vi "tape.fitness02_SS.vi"(2 "New Image":T2=refnum) -> ()   [LabVIEW 2013]
uses:
  <vilib>/vision/Image Controls.llb/IMAQ Image.ctl
  <vilib>/vision/NI_Vision_Development_Module.lvlib
panel:
  out "x/y 2":sgl
  out "x/y":sgl
  out "Waveform Chart 4":sgl(graph)=1.0503659
  out "In Range? 2":bool=TRUE
  in  "upper limit 2":sgl=1.1
  in  "lower  limit 2":sgl=0.9
  in  "Boolean":bool
  in  "Settings 2":T1={"Contrast"=170, "Filter width"=4, "Steepness"=50, "Subsampling Ratio"=10.0, "Scan Direction"=1, "Show Search Area"=TRUE, "Show Search Lines"=FALSE, "Show Edges Found"=TRUE, "Show Result"=TRUE} {"Scan Direction" items=["Outside to Inside", "Inside to Outside"]}
  in  "shot number":i16
  in  "lower  limit":sgl=0.9
  in  "upper limit":sgl=1.1
  out "In Range?":bool=TRUE
  out "Waveform Chart 3":sgl(graph)=1.0234288
  out "Y Graph":cluster{i16, "Y":sgl}[](graph)=[{1, "Y"=174.77158}, {1, "Y"=173.48274}, {1, "Y"=268.76178}, {1, "Y"=279.66354}]
  out "X Graph":cluster{i16, "X":sgl}[](graph)=[{1, "X"=246.72554}, {1, "X"=149.21423}, {1, "X"=152.1977}, {1, "X"=252.06}]
  out "tape status":bool=TRUE
  out "XY Graph":cluster{"X":sgl, "Y":sgl}[](graph)=[{"X"=246.72554, "Y"=174.77158}, {"X"=149.21423, "Y"=173.48274}, {"X"=152.1977, "Y"=268.76178}, {"X"=252.06, "Y"=279.66354}]
  out "Radius":dbl=52.693813240488524
  in  "Location of structure":T3={"Center X"=198, "Center Y"=228, "Inner Radius"=0, "Outer Radius"=210, "Start Angle"=0.0, "End Angle"=0.0} {"End Angle" format="%.2f"; "Start Angle" format="%.2f"; "Center X" scale=0.0..1024.0}
  in  "Settings":T1={"Contrast"=170, "Filter width"=4, "Steepness"=9, "Subsampling Ratio"=10.0, "Scan Direction"=1, "Show Search Area"=TRUE, "Show Search Lines"=FALSE, "Show Edges Found"=TRUE, "Show Result"=TRUE} {"Scan Direction" items=["Outside to Inside", "Inside to Outside"]}
  in  "input anulus 2":T3={"Center X"=173, "Center Y"=143, "Inner Radius"=0, "Outer Radius"=57, "Start Angle"=0.0, "End Angle"=0.0} {"End Angle" min=-90.0 max=90.0 step=1.0 format="%.2f"; "Start Angle" min=-90.0 max=90.0 step=1.0 format="%.2f"; "Center X" scale=0.0..1024.0}
  out "Image":T2(plugin-control)
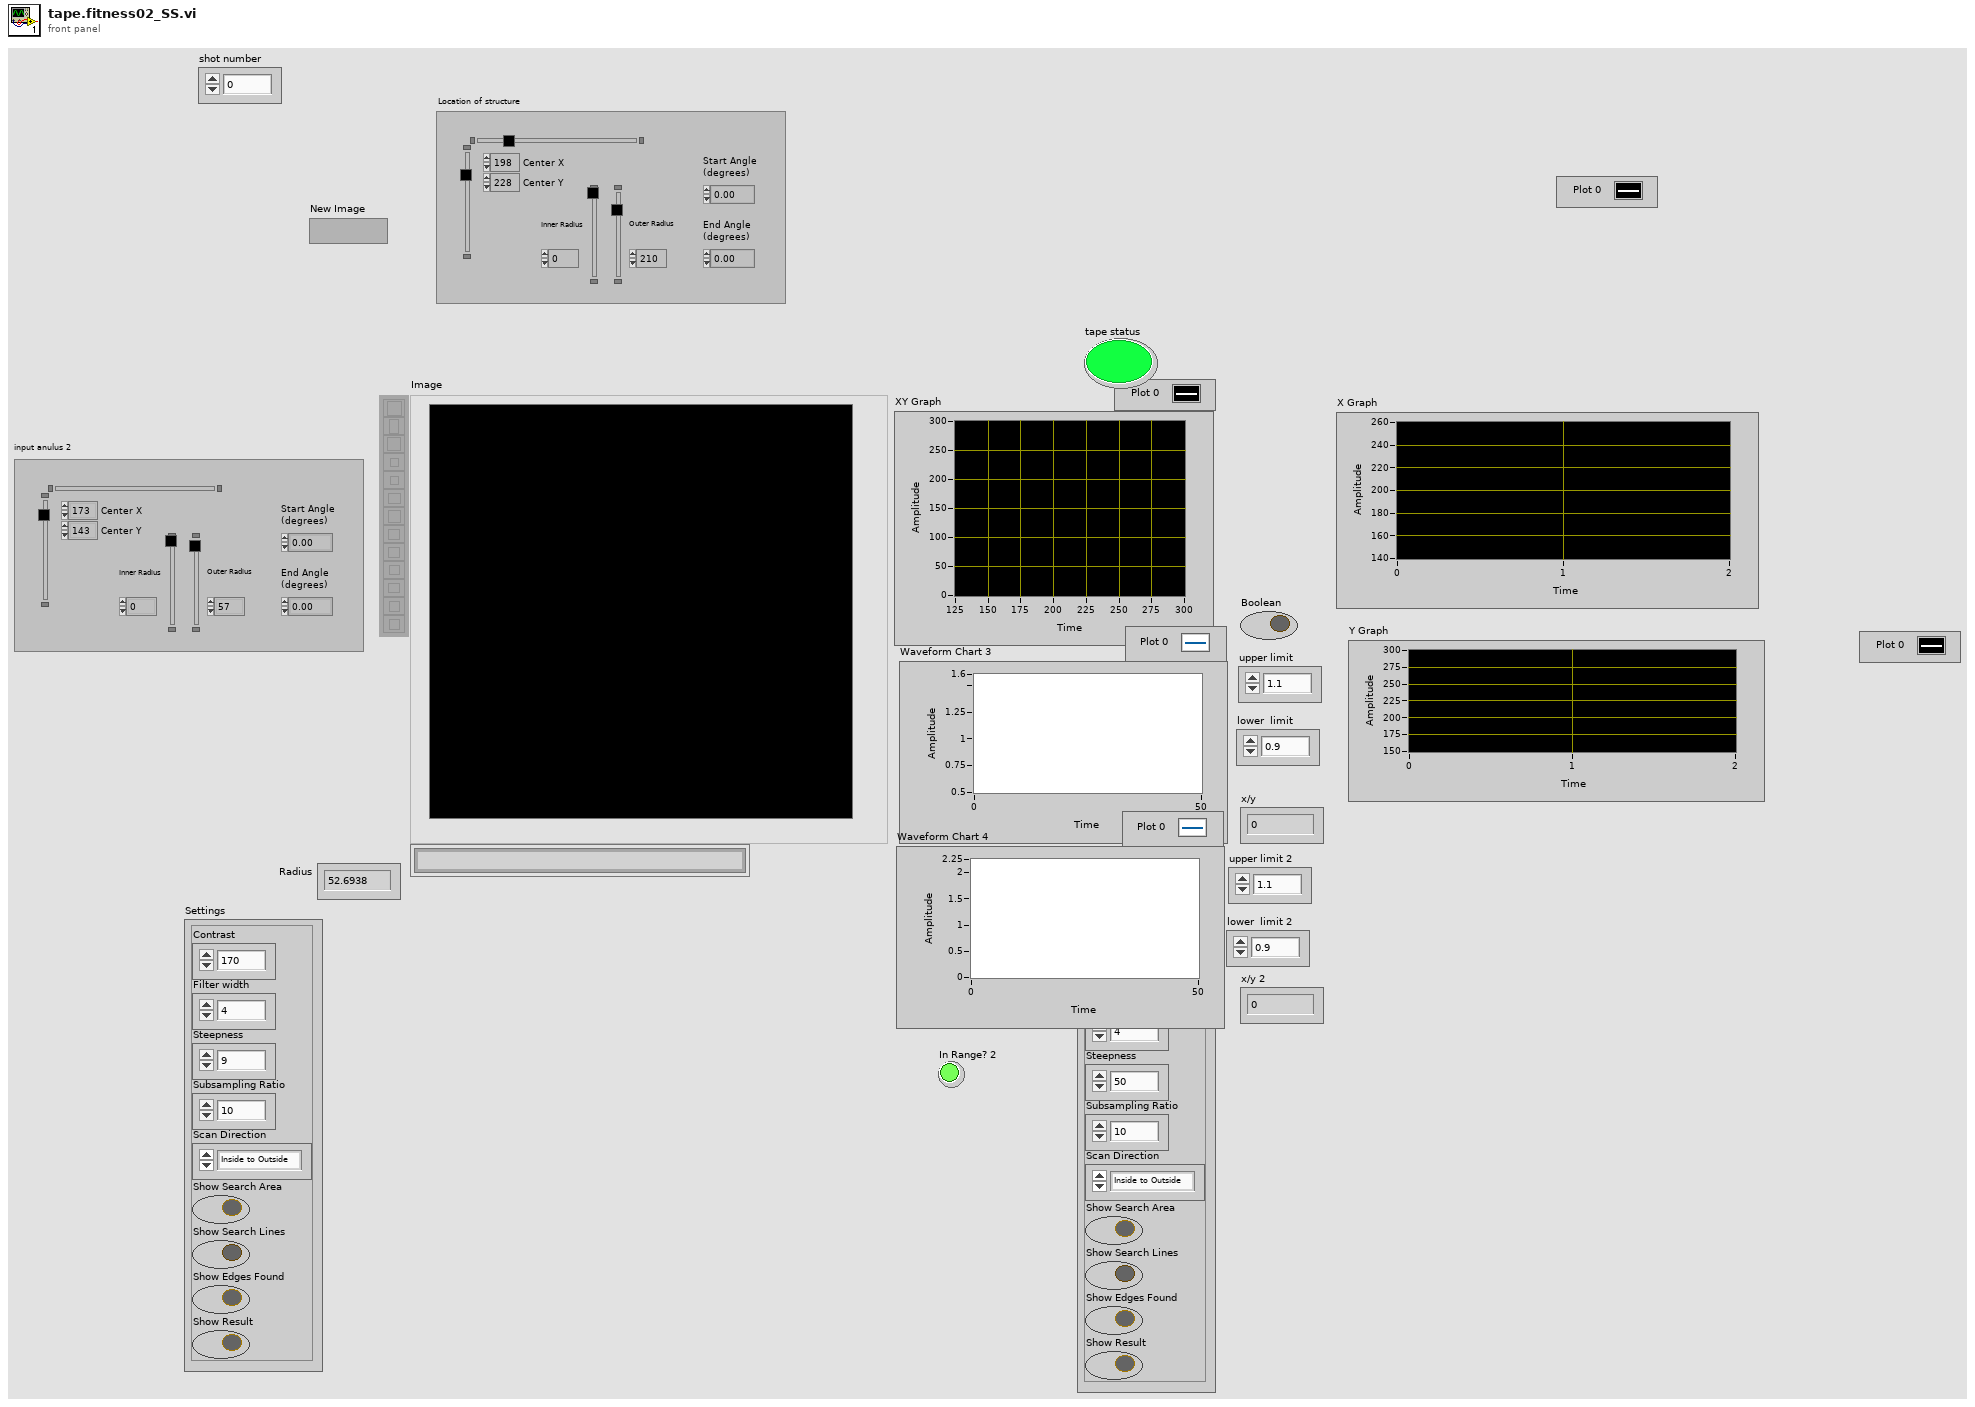
[diagram p1: front panel]
types:
  T1 = cluster{"Contrast":i32, "Filter width":i32, "Steepness":i32, "Subsampling Ratio":dbl, "Scan Direction":u32, "Show Search Area":bool, "Show Search Lines":bool, "Show Edges Found":bool, "Show Result":bool}
  T2 = typedef "IMAQ Image.ctl" = refnum<image>
  T3 = typedef "IMAQ Circle" = cluster{"Center X":i32, "Center Y":i32, "Inner Radius":i32, "Outer Radius":i32, "Start Angle":dbl, "End Angle":dbl}
  T4 = cluster{"Global Rectangle":i32[], "Contours":cluster{"Contour Type":u32, "ROI Type":u32, "Points":i32[]}[]}
  T5 = cluster{"Contour Type":u32, "ROI Type":u32, "Points":i32[]}[]
  T6 = cluster{"Contour Type":u32, "ROI Type":u32, "Points":i32[]}
  T7 = cluster{"Center":cluster{"X":sgl, "Y":sgl}, "Radius":dbl}
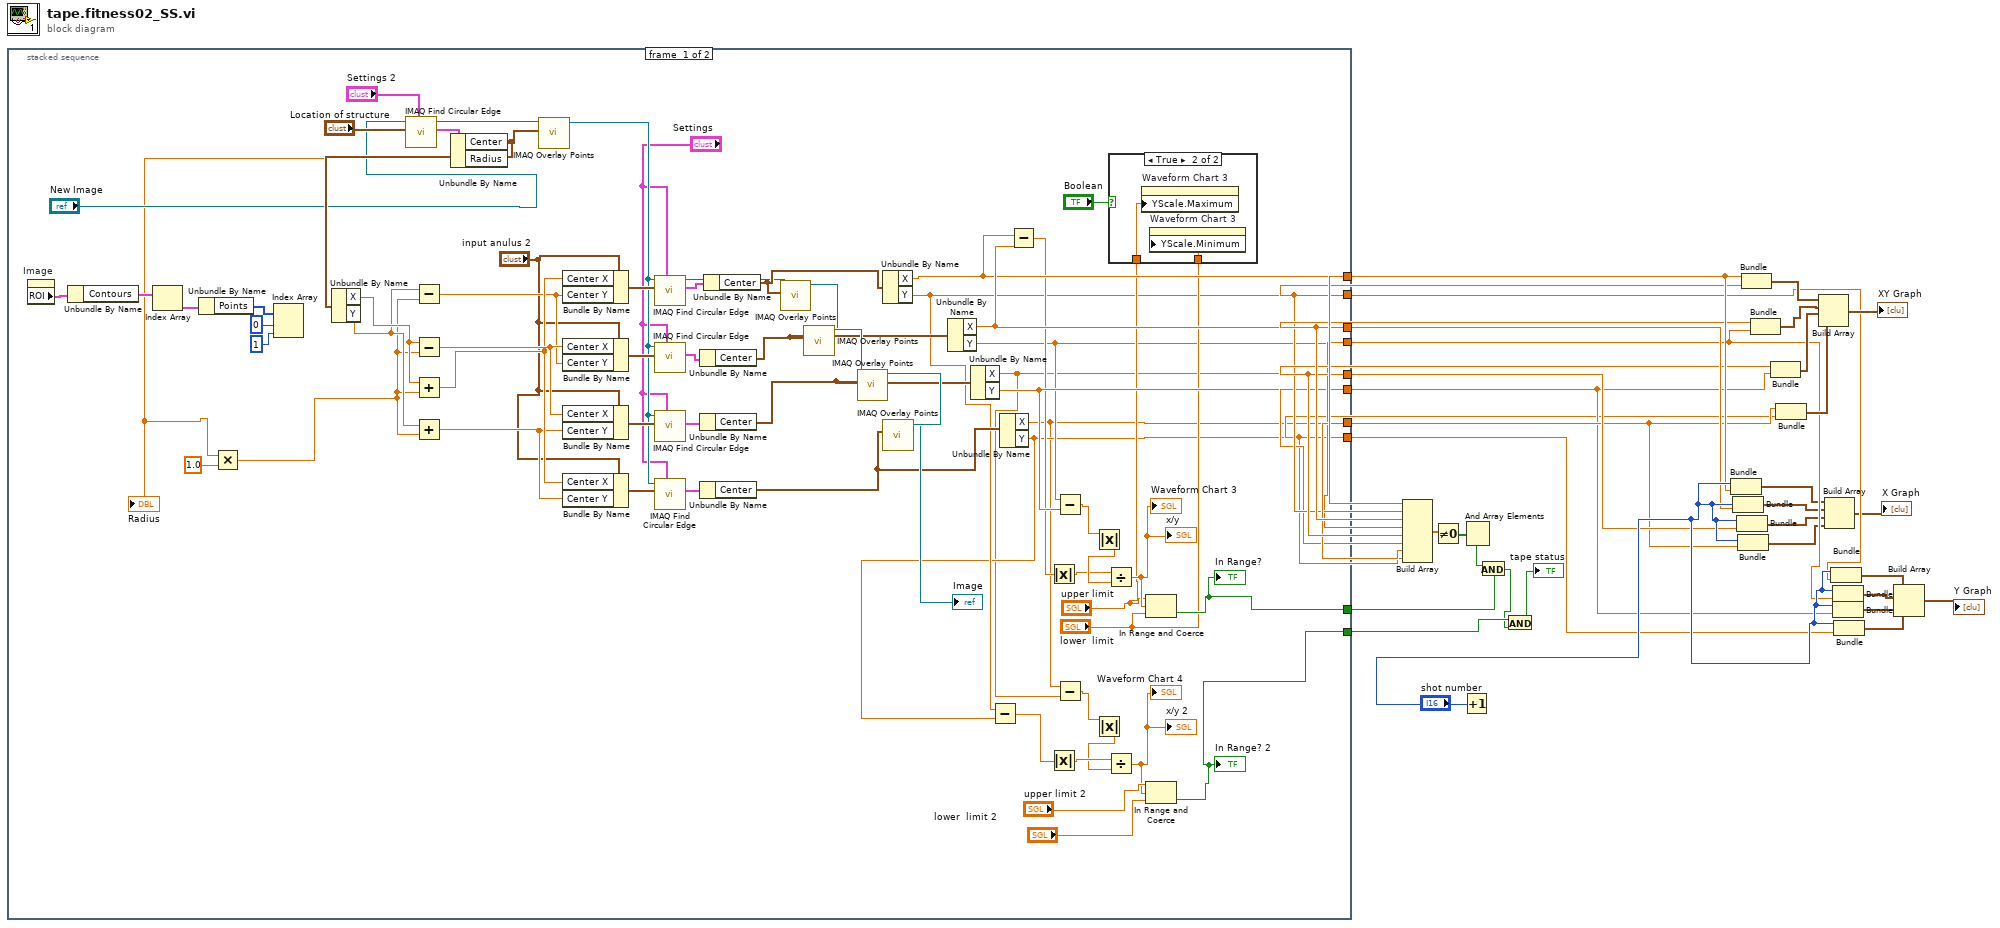
[diagram p0: block diagram]
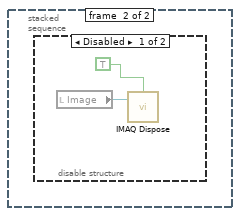
[diagram p3: hidden frame]
diagram:
  n1 = stacked-sequence {
    tunnel: [w60 _] -> w26
    tunnel: [w36 _] -> w22
    tunnel: [w61 _] -> w25
    tunnel: [w37 _] -> w21
    tunnel: [w33 _] -> w24
    tunnel: [w59 _] -> w20
    tunnel: [w34 _] -> w23
    tunnel: [w35 _] -> w19
    tunnel: [w53 _] -> w3
    tunnel: [w38 _] -> w4
    frame #0 {
      n2 = property on="Image" class="ImageControl"() -> ("ROI"=w92:T4)  [unwired: 2 in, 2 out]
      n3 = Unbundle By Name(w92) -> ("Contours"=w91:T5)
      n4 = Index Array(array=w91) -> (element=w90:T6)  [unwired: 1 in]
      n5 = Unbundle By Name(w90) -> ("Points"=w89:i32[])
      n6 = Index Array(array=w89, index #1=0 ("index"), index #2=1 ("index")) -> ()  [unwired: 2 out]
      n7 = call "IMAQ Find Circular Edge"("Settings"="Settings 2", "Circle or Annulus"="Location of structure", "Image"="New Image") -> ("Best Circle"=w78:T7, "Image Out"=w74:T2)  [unwired: 3 in, 4 out]
      n8 = Unbundle By Name(w78) -> ("Center"=w73:cluster{"X":sgl, "Y":sgl}, "Radius"=w47:dbl)
      "Radius" <- w47
      n9 = Multiply(x=w47, y=1.0) -> (x*y=w69:dbl)
      n10 = Unbundle By Name(w73) -> ("X"=w72:sgl, "Y"=w71:sgl)
      n11 = Subtract(x=w71, y=w69) -> (x-y=w83:dbl)
      n12 = Subtract(x=w72, y=w69) -> (x-y=w86:dbl)
      n13 = Add(x=w72, y=w69) -> (x+y=w85:dbl)
      n14 = Add(x=w71, y=w69) -> (x+y=w84:dbl)
      n15 = call "IMAQ Overlay Points"("Point"=w73, "Image"=w74) -> ("Image Out"=w77:T2)  [unwired: 8 in, 1 out]
      n16 = Bundle By Name(cluster="input anulus 2", "Center X"=w85, "Center Y"=w83) -> (w81:T3)
      n17 = Bundle By Name(cluster="input anulus 2", "Center X"=w86, "Center Y"=w83) -> (w82:T3)
      n18 = Bundle By Name(cluster="input anulus 2", "Center X"=w86, "Center Y"=w84) -> (w80:T3)
      n19 = Bundle By Name(cluster="input anulus 2", "Center X"=w85, "Center Y"=w84) -> (w79:T3)
      n20 = call "IMAQ Find Circular Edge"("Settings"="Settings", "Circle or Annulus"=w81, "Image"=w77) -> ("Best Circle"=w97:T7, "Image Out"=w66:T2)  [unwired: 3 in, 4 out]
      n21 = call "IMAQ Find Circular Edge"("Settings"="Settings", "Circle or Annulus"=w82, "Image"=w77) -> ("Best Circle"=w98:T7)  [unwired: 3 in, 5 out]
      n22 = call "IMAQ Find Circular Edge"("Settings"="Settings", "Circle or Annulus"=w80, "Image"=w77) -> ("Best Circle"=w96:T7)  [unwired: 3 in, 5 out]
      n23 = call "IMAQ Find Circular Edge"("Settings"="Settings", "Circle or Annulus"=w79, "Image"=w77) -> ("Best Circle"=w95:T7)  [unwired: 3 in, 5 out]
      n24 = Unbundle By Name(w98) -> ("Center"=w64:cluster{"X":sgl, "Y":sgl})
      n25 = Unbundle By Name(w96) -> ("Center"=w63:cluster{"X":sgl, "Y":sgl})
      n26 = Unbundle By Name(w95) -> ("Center"=w62:cluster{"X":sgl, "Y":sgl})
      n27 = Unbundle By Name(w97) -> ("Center"=w68:cluster{"X":sgl, "Y":sgl})
      n28 = call "IMAQ Overlay Points"("Point"=w68, "Image"=w66) -> ("Image Out"=w65:T2)  [unwired: 8 in, 1 out]
      n29 = call "IMAQ Overlay Points"("Point"=w64, "Image"=w65) -> ("Image Out"=w67:T2)  [unwired: 8 in, 1 out]
      n30 = call "IMAQ Overlay Points"("Point"=w63, "Image"=w67) -> ("Image Out"=w94:T2)  [unwired: 8 in, 1 out]
      n31 = Unbundle By Name(w68) -> ("X"=w60:sgl, "Y"=w36:sgl)
      n32 = call "IMAQ Overlay Points"("Point"=w62, "Image"=w94) -> ("Image Out"=→"Image":T2)  [unwired: 8 in, 1 out]
      n33 = Unbundle By Name(w64) -> ("X"=w61:sgl, "Y"=w37:sgl)
      n34 = Unbundle By Name(w63) -> ("X"=w33:sgl, "Y"=w59:sgl)
      n35 = Unbundle By Name(w62) -> ("X"=w34:sgl, "Y"=w35:sgl)
      n36 = Subtract(x=w36, y=w35) -> (x-y=w39:sgl)
      n37 = Subtract(x=w60, y=w61) -> (x-y=w55:sgl)
      n38 = Absolute Value(x=w55) -> (abs(x)=w54:sgl)
      n39 = Absolute Value(x=w39) -> (abs(x)=w43:sgl)
      n40 = Subtract(x=w37, y=w59) -> (x-y=w57:sgl)
      n41 = Subtract(x=w34, y=w33) -> (x-y=w41:sgl)
      n42 = Absolute Value(x=w57) -> (abs(x)=w56:sgl)
      n43 = Absolute Value(x=w41) -> (abs(x)=w42:sgl)
      n44 = Divide(x=w54, y=w56) -> (x/y=w58:sgl)
      "Waveform Chart 3" <- w58
      "x/y" <- w58
      n45 = Divide(x=w43, y=w42) -> (x/y=w40:sgl)
      "Waveform Chart 4" <- w40
      "x/y 2" <- w40
      n46 = case shown="True" "Boolean" {
        tunnel: "upper limit" -> [_ w100]
        tunnel: "lower  limit" -> [_ w99]
        frame False {
        }
        frame True {
          n47 = property on="Waveform Chart 3" class="WFChart (strict)"("YScale.Maximum"=w100) -> ()  [unwired: 2 in, 2 out]
          n48 = property on="Waveform Chart 3" class="WFChart (strict)"("YScale.Minimum"=w99) -> ()  [unwired: 2 in, 2 out]
        }
      }
      n49 = In Range and Coerce(upper limit="upper limit", x=w58, lower limit="lower  limit") -> (In Range?=w53:bool)  [unwired: 1 out]
      "In Range?" <- w53
      n50 = In Range and Coerce(upper limit="upper limit 2", x=w40, lower limit="lower  limit 2") -> (In Range?=w38:bool)  [unwired: 1 out]
      "In Range? 2" <- w38
    }
    frame #1 {
      n51 = disable-structure shown="Disabled" {
        frame Disabled {
          n52 = local read "Image"() -> (w102:T2)
          n53 = call "IMAQ Dispose"("All Images? (No)"=TRUE, "Image"=w102) -> ()  [unwired: 4 in, 1 out]
        }
        frame Enabled {
        }
      }
    }
  }
  n54 = Build Array(w26, w22, w25, w21, w24, w20, w23, w19) -> (w8:sgl[])
  n55 = Not Equal To 0?(x=w8) -> (x != 0?=w7:bool[])
  n56 = Increment(x="shot number") -> (x+1=w27:i16)
  n57 = And Array Elements(Boolean array=w7) -> (logical AND=w6:bool)
  n58 = And(x=w6, y=w3) -> (x .and. y?=w2:bool)
  n59 = And(x=w4, y=w2) -> (x .and. y?=→"tape status":bool)
  n60 = Bundle(w27, "X"=w26) -> (w18:cluster{i16, "X":sgl})  [unwired: 1 in]
  n61 = Bundle(w27, "X"=w25) -> (w17:cluster{i16, "X":sgl})  [unwired: 1 in]
  n62 = Bundle(w27, "X"=w24) -> (w16:cluster{i16, "X":sgl})  [unwired: 1 in]
  n63 = Bundle(w27, "X"=w23) -> (w15:cluster{i16, "X":sgl})  [unwired: 1 in]
  n64 = Bundle("X"=w26, "Y"=w22) -> (w32:cluster{"X":sgl, "Y":sgl})  [unwired: 1 in]
  n65 = Bundle("X"=w25, "Y"=w21) -> (w31:cluster{"X":sgl, "Y":sgl})  [unwired: 1 in]
  n66 = Bundle("X"=w24, "Y"=w20) -> (w30:cluster{"X":sgl, "Y":sgl})  [unwired: 1 in]
  n67 = Bundle("X"=w23, "Y"=w19) -> (w29:cluster{"X":sgl, "Y":sgl})  [unwired: 1 in]
  n68 = Build Array(w32, w31, w30, w29) -> (→"XY Graph":cluster{"X":sgl, "Y":sgl}[])
  n69 = Build Array(w18, w17, w16, w15) -> (→"X Graph":cluster{i16, "X":sgl}[])
  n70 = Bundle(w27, "Y"=w22) -> (w14:cluster{i16, "Y":sgl})  [unwired: 1 in]
  n71 = Bundle(w27, "Y"=w21) -> (w13:cluster{i16, "Y":sgl})  [unwired: 1 in]
  n72 = Bundle(w27, "Y"=w20) -> (w12:cluster{i16, "Y":sgl})  [unwired: 1 in]
  n73 = Bundle(w27, "Y"=w19) -> (w11:cluster{i16, "Y":sgl})  [unwired: 1 in]
  n74 = Build Array(w14, w13, w12, w11) -> (→"Y Graph":cluster{i16, "Y":sgl}[])
